vi "AIT 664 - ReadWrite LoopStats.vi"(0 "RT Data in":T2 {"End System Handle" format="%x"; "Label Transfer Config"."Block Data Refs"."Data Reference" format="%.0x"; "Status Config"."Hardware Out Dur Reference" format="%.0x"; "Status Config"."Hardware In Dur Reference" format="%.0x"; "Status Config"."Hardware Out Count Reference" format="%.0x"; "Status Config"."Hardware In Count Reference" format="%.0x"; "Status Config"."Error Data Reference" format="%.0x"; "Hardware Output Tx Channels"."Message Settings"."Transmit Channel Data Reference" format="%.0x"; "Hardware Output Tx Channels"."Message Settings"."Queue Transmit Channel" format="%.0x"; "Hardware Output Tx Channels"."Message Settings"."Driver Data"."Num Bits" min=1 max=32; "Hardware Output Tx Channels"."Message Settings"."Block Data Refs"."Data Reference" format="%.0x"; "Hardware Output Tx Channels"."Rx Com Udp Port"."Handle" format="%08x"; "Hardware Output Tx Channels"."Tx Com Udp Port"."Handle" format="%08x"; "Hardware Input Rx Channels"."Message Settings"."Transmit Channel Data Reference" format="%.0x"; "Hardware Input Rx Channels"."Message Settings"."Queue Transmit Channel" format="%.0x"; "Hardware Input Rx Channels"."Message Settings"."Driver Data"."Num Bits" min=1 max=32; "Hardware Input Rx Channels"."Message Settings"."Block Data Refs"."Data Reference" format="%.0x"; "Hardware Input Rx Channels"."Rx Com Udp Port"."Handle" format="%08x"; "Hardware Input Rx Channels"."Tx Com Udp Port"."Handle" format="%08x"}, 1 "Mode":T1, 3 "Late":bool, 11 "error in (no error)":errorcluster, 12 "Iteration Duration":i64) -> (4 "RT Data out":T2 {"End System Handle" format="%x"; "Label Transfer Config"."Block Data Refs"."Data Reference" format="%.0x"; "Status Config"."Hardware Out Dur Reference" format="%.0x"; "Status Config"."Hardware In Dur Reference" format="%.0x"; "Status Config"."Hardware Out Count Reference" format="%.0x"; "Status Config"."Hardware In Count Reference" format="%.0x"; "Status Config"."Error Data Reference" format="%.0x"; "Hardware Output Tx Channels"."Message Settings"."Transmit Channel Data Reference" format="%.0x"; "Hardware Output Tx Channels"."Message Settings"."Queue Transmit Channel" format="%.0x"; "Hardware Output Tx Channels"."Message Settings"."Driver Data"."Num Bits" min=1 max=32; "Hardware Output Tx Channels"."Message Settings"."Block Data Refs"."Data Reference" format="%.0x"; "Hardware Output Tx Channels"."Rx Com Udp Port"."Handle" format="%08x"; "Hardware Output Tx Channels"."Tx Com Udp Port"."Handle" format="%08x"; "Hardware Input Rx Channels"."Message Settings"."Transmit Channel Data Reference" format="%.0x"; "Hardware Input Rx Channels"."Message Settings"."Queue Transmit Channel" format="%.0x"; "Hardware Input Rx Channels"."Message Settings"."Driver Data"."Num Bits" min=1 max=32; "Hardware Input Rx Channels"."Message Settings"."Block Data Refs"."Data Reference" format="%.0x"; "Hardware Input Rx Channels"."Rx Com Udp Port"."Handle" format="%08x"; "Hardware Input Rx Channels"."Tx Com Udp Port"."Handle" format="%08x"}, 15 "error out":errorcluster)   [LabVIEW 2013, in "AIT 664 Custom Device.lvlib"]
uses:
  AIT 664 Custom Device.lvlib
  RT Controls/AIT 664  - RT Data.ctl
  RT Controls/AIT 664 - RT Hardware Channel.ctl
  RT Controls/AIT 664 - RT Message Settings.ctl
  <vilib>/NI Veristand/Custom Device API/Block Data Reference.ctl
  <vilib>/NI Veristand/Custom Device API/Data Reference.ctl
  RT Controls/AIT 664 - Driver Data.ctl
  Controls and Global/Start Bit.ctl
  Controls and Global/Number of Bits.ctl
  <vilib>/NI Veristand/Custom Device API/Custom Device Item Ref.ctl
  <userlib>/ARINC 664/AIT 664 Controls/General/Message Port.ctl
  <userlib>/ARINC 664/AIT 664 Controls/General/Direction.ctl
  <userlib>/ARINC 664/AIT 664 Controls/General/Message Port Type.ctl
  System Explorer/Controls/664 - Sampling Type.ctl
  RT Controls/Status Channels Config.ctl
  RT Controls/FIFO.ctl
  RT Controls/Label Transfer Config.ctl
  RT Controls/ReadWrite Selector.ctl
  <vilib>/NI Veristand/Custom Device API/Global Data Refs.vi
  <vilib>/NI Veristand/Custom Device API/Custom Device API.lvlib
  <userlib>/ARINC 664/AIT 664 API.lvlib
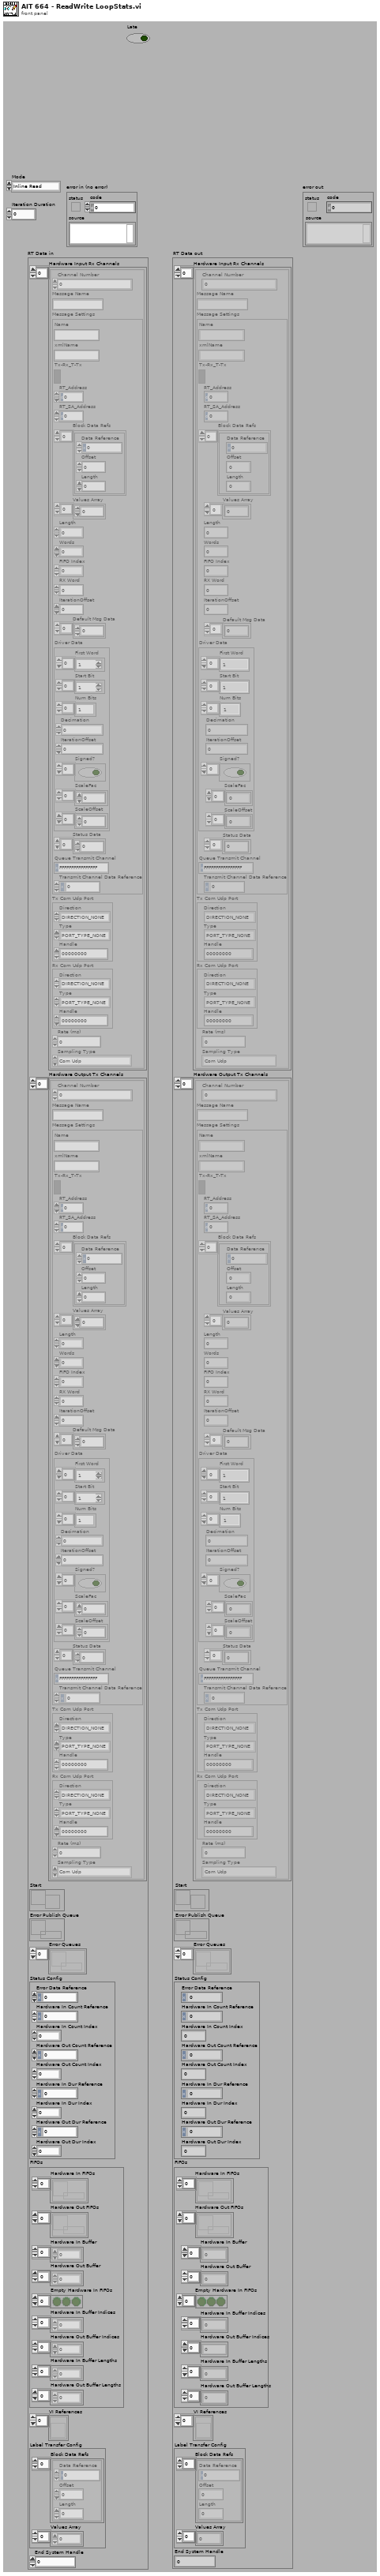
[diagram p1: front panel]
types:
  T1 = typedef "AIT 664 Custom Device.lvlib/ReadWrite Selector.ctl" = enum16{"Inline Read", "Inline Write", "Async HWIn", "Async HWOut"}
  T2 = typedef "AIT 664 Custom Device.lvlib/AIT 664  - RT Data.ctl" = cluster{"Hardware Input Rx Channels":T3[], "Hardware Output Tx Channels":T3[], "Start":refnum<notifier>, "Error Publish Queue":refnum<queue>, "Error Queues":refnum<queue>[], "Status Config":T15, "FIFOs":T16, "VI References":refnum<vi>[], "Label Transfer Config":T17, "End System Handle ":u64}
  T3 = typedef "AIT 664 Custom Device.lvlib/AIT 664 - RT Hardware Channel.ctl" = cluster{"Channel Number":u16, "Message Name":string, "Message Settings":T4, "Tx Com Udp Port":T11, "Rx Com Udp Port":T11, "Rate (ms)":u32, "Sampling Type":T14}
  T4 = typedef "AIT 664 Custom Device.lvlib/AIT 664 - RT Message Settings.ctl" = cluster{"Name":string, "xmlName":string, "Tx-Rx_T-Tx":bool, "RT_Address":u8, "RT_SA_Address":u8, "Block Data Refs":T5[], "Values Array":dbl[], "Length":i32, "Words":i32, "FIFO Index":i32, "RX Word":u32, "IterationOffset":i32, "Default Msg Data":u8[], "Driver Data":T7, "Status Data":u32[], "Queue Transmit Channel":T10, "Transmit Channel Data Reference":T6}
  T5 = typedef "Custom Device API.lvlib/Block Data Reference.ctl" = cluster{"Data Reference":T6, "Offset":i32, "Length":i32}
  T6 = typedef "Custom Device API.lvlib/Data Reference.ctl" = i32
  T7 = typedef "AIT 664 Custom Device.lvlib/AIT 664 - Driver Data.ctl" = cluster{"First Word":T8[], "Start Bit":T8[], "Num Bits":T9[], "Decimation":i32, "IterationOffset":i32, "Signed?":bool[], "ScaleFac":dbl[], "ScaleOffset":dbl[]}
  T8 = typedef "AIT 664 Custom Device.lvlib/Start Bit.ctl" = i32
  T9 = typedef "AIT 664 Custom Device.lvlib/Number of Bits.ctl" = i32
  T10 = typedef "Custom Device API.lvlib/Custom Device Item Ref.ctl" = u64
  T11 = typedef "AIT 664 API.lvlib/Message Port.ctl" = cluster{"Direction":T12, "Type":T13, "Handle":u64}
  T12 = typedef "AIT 664 API.lvlib/Direction.ctl" = enum16{"DIRECTION_NONE", "DIRECTION_TX", "DIRECTION_RX"}
  T13 = typedef "AIT 664 API.lvlib/Message Port Type.ctl" = enum16{"PORT_TYPE_NONE", "COM_UDP", "SAP_UDP", "SAP_IP", "SAP_MAC", "COTS_MAC", "COTS_MAC_RAW"}
  T14 = typedef "AIT 664 Custom Device.lvlib/664 - Sampling Type.ctl" = enum16{"Com Udp", "Com Udp Queuing", "Sap Udp", "Sap Ip", "Sap Mac", "Unknown"}
  T15 = typedef "AIT 664 Custom Device.lvlib/Status Channels Config.ctl" = cluster{"Error Data Reference":T6, "Hardware In Count Reference":T6, "Hardware In Count Index":i32, "Hardware Out Count Reference":T6, "Hardware Out Count Index":i32, "Hardware In Dur Reference":T6, "Hardware In Dur Index":i32, "Hardware Out Dur Reference":T6, "Hardware Out Dur Index":i32}
  T16 = typedef "AIT 664 Custom Device.lvlib/FIFO.ctl" = cluster{"Hardware In FIFOs":refnum<k33>[], "Hardware Out FIFOs":refnum<k33>[], "Hardware In Buffer":dbl[], "Hardware Out Buffer":dbl[], "Empty Hardware In FIFOs":bool[], "Hardware In Buffer Indices":i32[], "Hardware Out Buffer Indices":i32[], "Hardware In Buffer Lengths":i32[], "Hardware Out Buffer Lengths":i32[]}
  T17 = typedef "AIT 664 Custom Device.lvlib/Label Transfer Config.ctl" = cluster{"Block Data Refs":T5[], "Values Array":dbl[]}
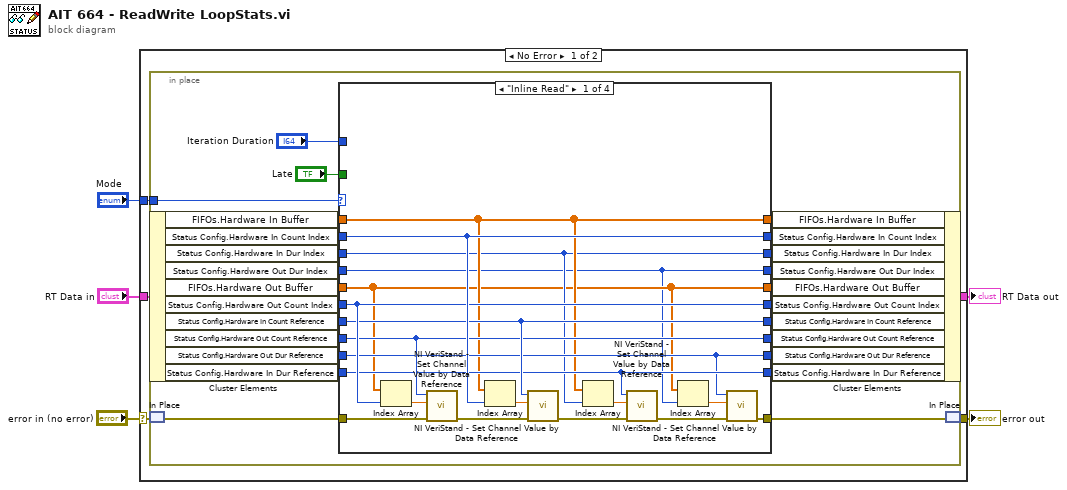
[diagram p0: block diagram]
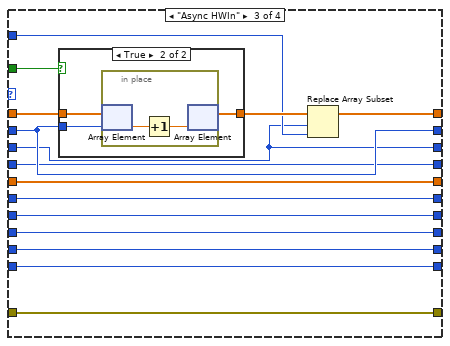
[diagram p3: hidden frame]
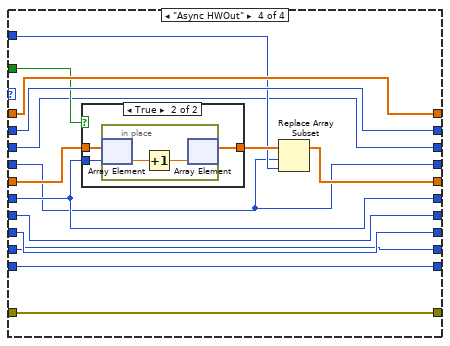
[diagram p5: hidden frame]
diagram:
  n1 = case shown="No Error" "error in (no error)" {
    selector: "error in (no error)" -> [w9 w109]
    tunnel: "RT Data in" -> [w10 w108]
    tunnel: [w8 w108] -> w3
    tunnel: [w7 w109] -> w2
    tunnel: "Mode" -> [w6 _]
    frame No Error {
      n2 = in-place {
        in-place-border: w6 -> [w27]
        n3 = in-place-cluster #1(w10) -> ("FIFOs.Hardware In Buffer"=w35:dbl[], "Status Config.Hardware In Count Index"=w34:i32, "Status Config.Hardware In Dur Index"=w23:i32, "Status Config.Hardware Out Dur Index"=w21:i32, "FIFOs.Hardware Out Buffer"=w33:dbl[], "Status Config.Hardware Out Count Index"=w32:i32, "Status Config.Hardware In Count Reference"=w29:T6, "Status Config.Hardware Out Count Reference"=w28:T6, "Status Config.Hardware Out Dur Reference"=w20:T6, "Status Config.Hardware In Dur Reference"=w19:T6)
        n4 = in-place-match #2(w9) -> (w31:errorcluster)
        n5 = case shown="\"Inline Read\"" w27 {
          tunnel: w35 -> [w41 w59 w74 w98]
          tunnel: w34 -> [w50 w60 w73 w97]
          tunnel: w33 -> [w37 w61 w80 w95]
          tunnel: w32 -> [w49 w62 w79 w94]
          tunnel: w31 -> [w54 w65 w76 w99]
          tunnel: [w45 w65 w76 w99] -> w30
          tunnel: w29 -> [w48 w63 w77 w100]
          tunnel: w28 -> [w47 w64 w78 w101]
          tunnel: [w47 w64 w78 w101] -> w15
          tunnel: [w48 w63 w77 w100] -> w14
          tunnel: [w49 w62 w79 w94] -> w26
          tunnel: [w37 w61 w80 w92] -> w25
          tunnel: [w50 w60 w73 w97] -> w11
          tunnel: [w41 w59 w71 w98] -> w18
          tunnel: "Late" -> [_ _ w75 w96]
          tunnel: w23 -> [w39 w57 w69 w90]
          tunnel: "Iteration Duration" -> [_ _ w70 w91]
          tunnel: [w39 w57 w69 w90] -> w12
          tunnel: [w36 w58 w68 w89] -> w13
          tunnel: w21 -> [w36 w58 w68 w89]
          tunnel: [w42 w56 w67 w88] -> w16
          tunnel: w20 -> [w42 w56 w67 w88]
          tunnel: [w43 w55 w66 w87] -> w17
          tunnel: w19 -> [w43 w55 w66 w87]
          frame "Inline Read" {
            n6 = Index Array(array=w37, index=w49) -> (element=w52:dbl)
            n7 = call <vilib>:"NI VeriStand - Set Channel Value by Data Reference.vi"("error in (no error)"=w54, "Value"=w52, "Data Reference in"=w47) -> ("error out"=w51:errorcluster)  [unwired: 8 in]
            n8 = Index Array(array=w41, index=w50) -> (element=w53:dbl)
            n9 = call <vilib>:"NI VeriStand - Set Channel Value by Data Reference.vi"("error in (no error)"=w51, "Value"=w53, "Data Reference in"=w48) -> ("error out"=w46:errorcluster)  [unwired: 8 in]
            n10 = Index Array(array=w41, index=w39) -> (element=w40:dbl)
            n11 = call <vilib>:"NI VeriStand - Set Channel Value by Data Reference.vi"("error in (no error)"=w46, "Value"=w40, "Data Reference in"=w43) -> ("error out"=w44:errorcluster)  [unwired: 8 in]
            n12 = Index Array(array=w37, index=w36) -> (element=w38:dbl)
            n13 = call <vilib>:"NI VeriStand - Set Channel Value by Data Reference.vi"("error in (no error)"=w44, "Value"=w38, "Data Reference in"=w42) -> ("error out"=w45:errorcluster)  [unwired: 8 in]
          }
          frame Default {
          }
          frame "Async HWIn" {
            n14 = case shown="True" w75 {
              tunnel: w74 -> [w81 w84]
              tunnel: w73 -> [_ w83]
              tunnel: [w81 w82] -> w72
              frame False {
              }
              frame True {
                n15 = in-place {
                  n16 = in-place-array #3(w84, w83) -> (w86:dbl)
                  n17 = Increment(x=w86) -> (x+1=w85:dbl)
                  n18 = in-place-array #3(w85) -> (w82:dbl[])  [unwired: 1 out]
                }
              }
            }
            n19 = Replace Array Subset(array=w72, new element=w70, index=w69) -> (w71:dbl[])
          }
          frame "Async HWOut" {
            n20 = case shown="True" w96 {
              tunnel: [w102 w105] -> w93
              tunnel: w95 -> [w102 w104]
              tunnel: w94 -> [_ w103]
              frame False {
              }
              frame True {
                n21 = in-place {
                  n22 = in-place-array #4(w104, w103) -> (w107:dbl)
                  n23 = Increment(x=w107) -> (x+1=w106:dbl)
                  n24 = in-place-array #4(w106) -> (w105:dbl[])  [unwired: 1 out]
                }
              }
            }
            n25 = Replace Array Subset(array=w93, new element=w91, index=w89) -> (w92:dbl[])
          }
        }
        n26 = in-place-cluster #1("FIFOs.Hardware In Buffer"=w18, "Status Config.Hardware In Count Index"=w11, "Status Config.Hardware In Dur Index"=w12, "Status Config.Hardware Out Dur Index"=w13, "FIFOs.Hardware Out Buffer"=w25, "Status Config.Hardware Out Count Index"=w26, "Status Config.Hardware In Count Reference"=w14, "Status Config.Hardware Out Count Reference"=w15, "Status Config.Hardware Out Dur Reference"=w16, "Status Config.Hardware In Dur Reference"=w17) -> (w8:T2)
        n27 = in-place-match #2(w30) -> (w7:errorcluster)
      }
    }
    frame Error {
    }
  }
  "error out" <- w2
  "RT Data out" <- w3
